vi "Main.vi"() -> ()   [LabVIEW 2016]
uses:
  Input_parameters.ctl
panel:
  in  "DMM device":T1(ring)
  out "Elapsed time":dbl format="%<%H:%M:%S>t"
  out "Estimated remaining time":dbl format="%<%H:%M:%S>t"
  in  "Sensor type":T2(ring)=enum."Diode"
  in  "Single channel?":bool=TRUE
  in  "Output file":refnum<k7>(container)
  in  "Scan voltages":string="10\n20"
  out "Current channel":dbl format="%#_13g"
  out "Current voltage (V)":dbl format="%#_13g"
  in  "Data storage location (def: ./results)":path
  in  "AcroPDF":refnum<k7>(container)
  in  "Plot after execution?":bool
  in  "Voltage limit (V)":dbl=1000.0
  in  "Compliance  level (uA)":dbl=100.0
  in  "VISA resource name LCR":refnum<visa-resource-name>="LCR_E4980A"
  in  "VISA resource name DMM":refnum<visa-resource-name>="DMM_2001"
  in  "VISA resource name source":refnum<visa-resource-name>="Source_2410"
  in  "Switch delay (s)":dbl
  in  "Voltage delay (s)":dbl=1.0
  in  "Display channel":i32=1
  in  "Open after execution?":bool
  in  "Identifier (eg. wafer number)":string="W311-D1_2s_135channels"
  in  "Measurement type":enum16{"IV", "CV", "Test"}(ring)=enum."Test"
  out "Single channel":cluster{"X":dbl[], "Y":dbl[]}[](graph) caption="XY Graph"
  out "Channels":cluster{i32[], dbl[]}[](graph) caption="XY Graph"
  in  "Stop":bool
  # "Ctrl+H for read mode"
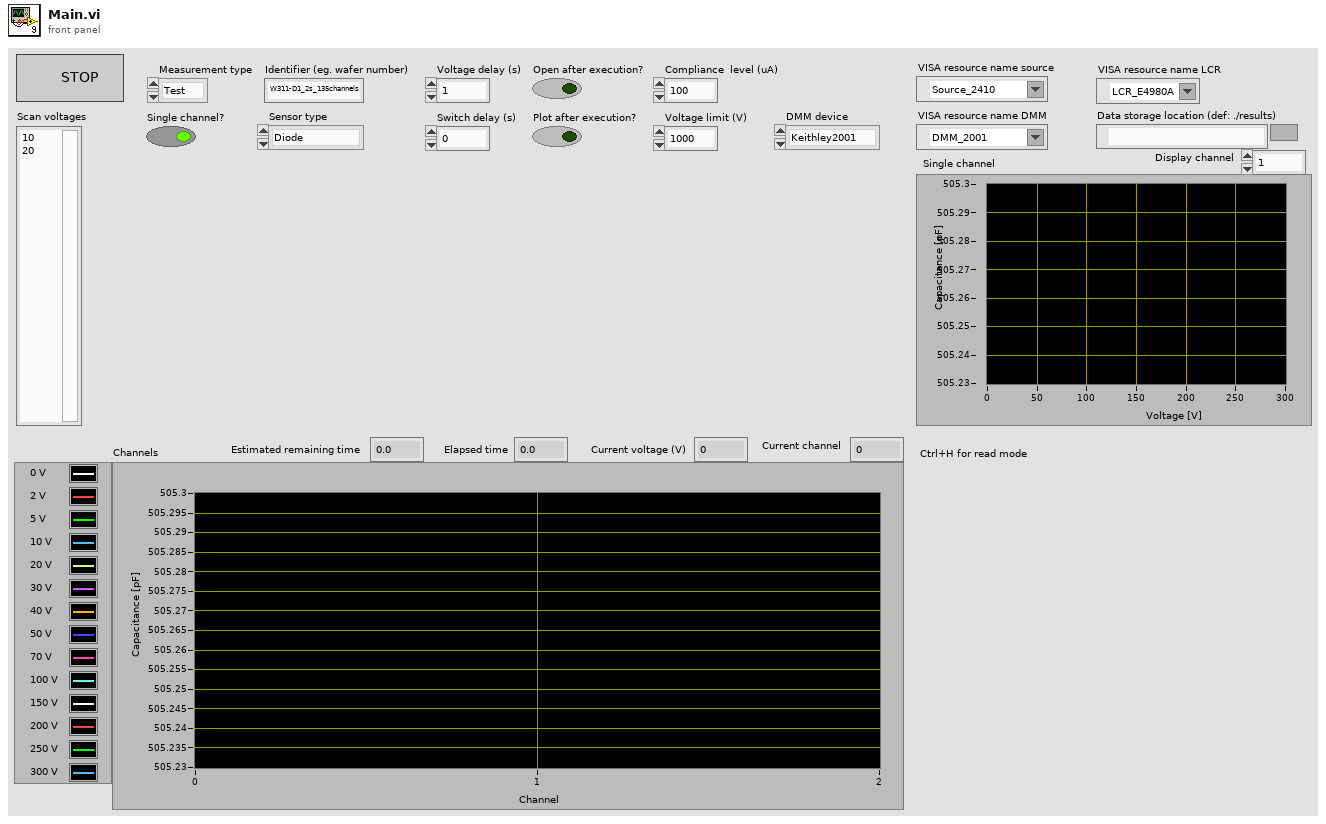
[diagram p1: front panel]
types:
  T1 = enum16{"Keithley2001", "Keithley2450", "Keithley2410"}
  T2 = enum16{"HPK_6in_135", "HPK_8in_256", "INF_8in_256", "Diode"}
  T3 = typedef "Input_parameters.ctl" = cluster{"Measurement type":enum16{"IV", "CV", "Test"}, "Sensor type":enum16{"HPK_6in_135", "HPK_8in_256", "INF_8in_256", "Diode"}, "Identifier":string, "Open after execution?":bool, "Plot after execution?":bool, "Display channel":i32, "Voltage Delay (s)":dbl, "Switch Delay (s)":dbl, "VISA resource name source":refnum<visa-resource-name>, "VISA resource name DMM":refnum<visa-resource-name>, "VISA resource name LCR":refnum<visa-resource-name>, "Compliance  Level (uA)":dbl, "Voltage Limit (V)":dbl, "Data storage location":string, "Scan voltages":string, "Use source as DMM?":bool, "Single channel?":bool, "LCR signal frequenzy (Hz)":dbl, "DMM device":enum16{"Keithley2001", "Keithley2450", "Keithley2410"}}
  T4 = typedef "Dynamic_data.ctl" = cluster{"Output file":path, "Y-label text":string, "Current set voltage":dbl, "Set voltage column":dbl[], "Pad number column":dbl[], "Data  column":dbl[], "Number of voltages":i32, "Compliance current (A)":dbl, "Geofile":string, "Peak voltage":dbl, "Hex PDF file":string, "Voltage array":dbl[], "Total current column":dbl[], "Timestamp column":dbl[], "Data name":string, "Data unit":string, "2nd data column":dbl[], "2nd data name":string, "2nd data unit":string, "3rd data column":dbl[], "4th data column":dbl[], "3rd data name":string, "3rd data unit":string, "4th data name":string, "4th data unit":string, "Actual voltage column":dbl[]}
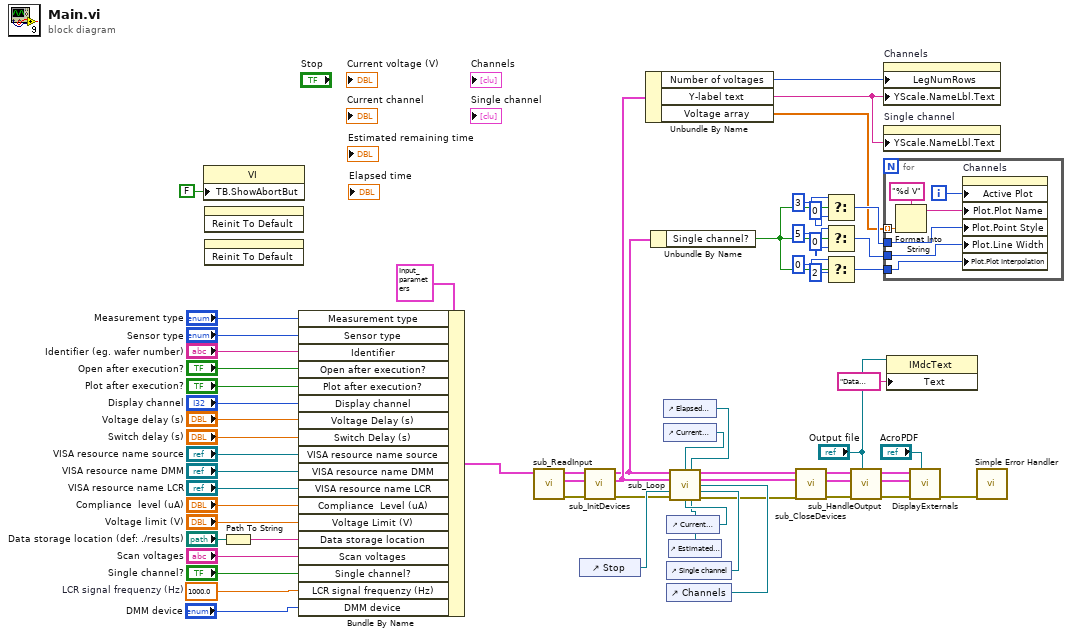
[diagram p0: block diagram]
diagram:
  w2 = 1000.0  # LCR signal frequenzy (Hz)
  n1 = property class="VI"("TB.ShowAbortBut"=FALSE ("Tool Bar:Show Abort Button")) -> ()  [unwired: 2 in, 2 out]
  n2 = invoke on="Stop" class="Bool (strict)" method="Reinit To Default"() -> ()  [unwired: 3 in, 3 out]
  n3 = invoke on="Single channel" class="XYGraph (strict)" method="Reinit To Default"() -> ()  [unwired: 3 in, 3 out]
  n4 = Path To String(path="Data storage location (def: ./results)") -> (string=w12:string)
  n5 = Bundle By Name(cluster=T3 {"Measurement type"=enum."Test", "Sensor type"=enum."HPK_6in_135", "Identifier"="test.txt", "Open after execution?"=FALSE, "Plot after execution?"=FALSE, "Display channel"=0, "Voltage Delay (s)"=0.5, "Switch Delay (s)"=0.01, "VISA resource name source"="", "VISA resource name DMM"="", "VISA resource name LCR"="", "Compliance  Level (uA)"=10.0, "Voltage Limit (V)"=1000.0, "Data storage location"="", "Scan voltages"="", "Use source as DMM?"=FALSE, "Single channel?"=FALSE, "LCR signal frequenzy (Hz)"=10.0, "DMM device"=enum."Keithley2001"} ("Input parameters 2"), "Measurement type"="Measurement type", "Sensor type"="Sensor type", "Identifier"="Identifier (eg. wafer number)", "Open after execution?"="Open after execution?", "Plot after execution?"="Plot after execution?", "Display channel"="Display channel", "Voltage Delay (s)"="Voltage delay (s)", "Switch Delay (s)"="Switch delay (s)", "VISA resource name source"="VISA resource name source", "VISA resource name DMM"="VISA resource name DMM", "VISA resource name LCR"="VISA resource name LCR", "Compliance  Level (uA)"="Compliance  level (uA)", "Voltage Limit (V)"="Voltage limit (V)", "Data storage location"=w12, "Scan voltages"="Scan voltages", "Single channel?"="Single channel?", "LCR signal frequenzy (Hz)"=w2, "DMM device"="DMM device") -> (w25:T3)
  n6 = call "sub_ReadInput.vi"("Input parameters"=w25) -> ("error out"=w60:errorcluster, "Dynamic data"=w57:T4, "Input parameters"=w61:T3)  [unwired: 8 in]
  n7 = control-ref of="Stop"() -> (w53:refnum<vi>)
  n8 = call "sub_InitDevices.vi"("error in (no error)"=w60, "Dynamic data"=w57, "Input parameters"=w61) -> ("error out"=w52:errorcluster, "Dynamic data"=w54:T4, "Input parameters"=w7:T3)  [unwired: 6 in]
  n9 = Unbundle By Name(w54) -> ("Number of voltages"=w55:i32, "Y-label text"=w44:string, "Voltage array"=w34:dbl[])
  n10 = Unbundle By Name(w7) -> ("Single channel?"=w6:bool)
  n11 = control-ref of="Elapsed time"() -> (w3:refnum<vi>)
  n12 = control-ref of="Current voltage (V)"() -> (w46:refnum<vi>)
  n13 = control-ref of="Current channel"() -> (w45:refnum<vi>)
  n14 = control-ref of="Single channel"() -> (w48:refnum<vi>)
  n15 = control-ref of="Channels"() -> (w49:refnum<vi>)
  n16 = control-ref of="Estimated remaining time"() -> (w4:refnum<vi>)
  n17 = call "sub_Loop.vi"("Input parameters"=w7, "Current voltage"=w46, "Elapsed time"=w3, "Dynamic data"=w54, "Channels"=w49, "Stop"=w53, "Single channel"=w48, "error in (no error)"=w52, "Current channel"=w45, "Estimated remaining time"=w4) -> ("Input parameters"=w51:T3, "Dynamic data"=w50:T4, "error out"=w47:errorcluster)  [unwired: 3 in]
  n18 = call "sub_CloseDevices.vi"("error in (no error)"=w47, "Dynamic data"=w50, "Input parameters"=w51) -> ("error out"=w59:errorcluster, "Dynamic data"=w56:T4, "Input parameters"=w58:T3)  [unwired: 6 in]
  n19 = Select(t=u8 3 ("Plot.Point Style"), s=w6, f=u8 0 ("Plot.Point Style")) -> (s? t:f=w35:u8)
  n20 = Select(t=u8 5 ("Plot.Point Style"), s=w6, f=u8 0 ("Plot.Point Style")) -> (s? t:f=w36:u8)
  n21 = Select(t=u8 0 ("Plot.Point Style"), s=w6, f=u8 2 ("Plot.Point Style")) -> (s? t:f=w37:u8)
  n22 = call "sub_HandleOutput.vi"("Output file text box"="Output file", "error in (no error)"=w59, "Dynamic data"=w56, "Input parameters"=w58) -> ("error out"=w32:errorcluster, "Dynamic data"=w31:T4, "Input parameters"=w30:T3)  [unwired: 5 in]
  n23 = property on="Channels" class="XYGraph (strict)"("LegNumRows"=w55, "YScale.NameLbl.Text"=w44) -> ()  [unwired: 2 in, 2 out]
  n24 = property on="Single channel" class="XYGraph (strict)"("YScale.NameLbl.Text"=w44) -> ()  [unwired: 2 in, 2 out]
  n25 = for {
    tunnel: w37 -> [w67]
    tunnel: w36 -> [w66]
    tunnel: w35 -> [w65]
    tunnel: w34 -> [w62] mode=indexing
    i -> [w63]
    n26 = Format Into String(format string="%d V", w62) -> (resulting string=w68:string)  [unwired: 2 in, 1 out]
    n27 = property on="Channels" class="XYGraph (strict)"("Active Plot"=w63, "Plot.Plot Name"=w68, "Plot.Point Style"=w65, "Plot.Line Width"=w66, "Plot.Plot Interpolation"=w67) -> ()  [unwired: 2 in, 2 out]
  }
  n28 = property class="IMdcText"(reference="Output file", "Text"="Data taking in progress...") -> ()  [unwired: 1 in, 2 out]
  n29 = call "DisplayExternals.vi"("AcroPDF"="AcroPDF", "error in (no error)"=w32, "Dynamic data"=w31, "Input parameters"=w30) -> ("error out"=w33:errorcluster)  [unwired: 4 in, 3 out]
  n30 = call <vilib>:"Simple Error Handler.vi"("error in (no error)"=w33) -> ()  [unwired: 4 in, 5 out]
